vi "class_data.vi"() -> ()   [LabVIEW 2010, in "ImagingModeDL090130Frame.lvclass"]
uses:
  ImagingModeDL090130Frame.lvclass
  control_refs.ctl
panel:
  in  "control refs":T1
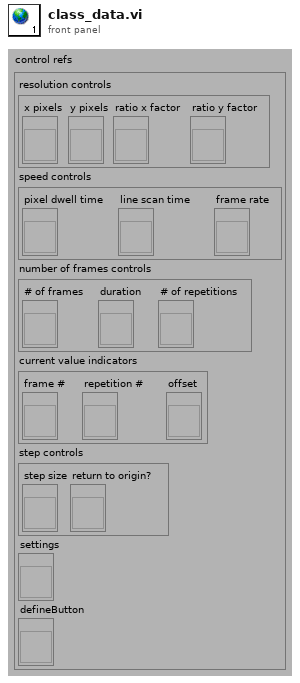
[diagram p1: front panel]
types:
  T1 = typedef "ImagingModeDL090130Frame.lvclass/control_refs.ctl" = cluster{"resolution controls":cluster{"x pixels":refnum<vi>, "y pixels":refnum<vi>, "ratio x factor":refnum<vi>, "ratio y factor":refnum<vi>}, "speed controls":cluster{"pixel dwell time":refnum<vi>, "line scan time":refnum<vi>, "frame rate":refnum<vi>}, "number of frames controls":cluster{"# of frames":refnum<vi>, "duration":refnum<vi>, "# of repetitions":refnum<vi>}, "current value indicators":cluster{"frame #":refnum<vi>, "repetition #":refnum<vi>, "offset":refnum<vi>}, "step controls":cluster{"step size":refnum<vi>, "return to origin?":refnum<vi>}, "settings":refnum<vi>, "defineButton":refnum<vi>}
diagram:
